vi "EstimateStates.vi"(8 "error in (no error)":errorcluster, 10 "Vessel in":refnum<class "Vessel.lvclass">, 11 "Kalman Filter in":refnum<class "Kalman Filter.lvclass">) -> (0 "error out":errorcluster, 2 "Vessel out":refnum<class "Vessel.lvclass">, 3 "Kalman Filter out":refnum<class "Kalman Filter.lvclass">)   [LabVIEW 2014, in "Observer Library.lvlib" / "Kalman Filter.lvclass"]
uses:
  Kalman Filter.lvclass
  ROV/Vessel.lvclass
  <vilib>/Analysis/Matrix/Numeric/Conversions/Matrix To Array - RM.vi
  <vilib>/imath/engines/lvmath2/RunTimeEngine/IndexRead/NIMS V(S).vi
  <instcachedir>/0/NIMS V(S)_0488751826AF41519A22953C041130DC.lvgen/NIMS V(S)_0488751826AF41519A22953C041130DC_000.vi
  <vilib>/imathl/engines/lvmath/Functions/Error Handling/Create Error.vi
  <vilib>/imath/engines/lvmath2/RunTimeEngine/IndexReplace/NIMS V(S)=S.vi
  <instcachedir>/0/NIMS V(S)=S_2D52C4EC15D8415E870AEE69FB516CCA.lvgen/NIMS V(S)=S_2D52C4EC15D8415E870AEE69FB516CCA_000.vi
  <vilib>/imath/engines/lvmath2/RunTimeEngine/BuiltInFunctions/mod/NIMS_mod_no_size_check.vi
  <instcachedir>/0/NIMS_mod_no_size_check_5393E3382FD241D281EEB71DA286C65B.lvgen/NIMS_mod_no_size_check_5393E3382FD241D281EEB71DA286C65B_001.vi
  <vilib>/imath/engines/lvmath2/RunTimeEngine/RangeToken/NIMS_Range.vi
  <instcachedir>/0/NIMS_Range_9BCE657718DF4976A877346C61F22738.lvgen/NIMS_Range_9BCE657718DF4976A877346C61F22738_000.vi
  <vilib>/imath/engines/lvmath2/RunTimeSupport/NIMS_Error if Not Equal.vi
  <instcachedir>/0/NIMS_Error if Not Equal_8A0E9F659B9142D69417CC259581C4FD.lvgen/NIMS_Error if Not Equal_8A0E9F659B9142D69417CC259581C4FD_001.vi
  <vilib>/imath/engines/lvmath2/RunTimeEngine/IndexRead/NIMS M(V,$).vi
  <instcachedir>/0/NIMS M(V,$)_21A5155762F74C04AE4EA67BEE0D3EF5.lvgen/NIMS M(V,$)_21A5155762F74C04AE4EA67BEE0D3EF5_004.vi
  <vilib>/imath/engines/lvmath2/RunTimeEngine/ErrorHandling/NIMS_Create Error From Enums.vi
  <vilib>/imath/engines/lvmath2/RunTimeEngine/ArithmeticOperatorToken/NIMS_ArithmeticOperator_multmx.vi
  <instcachedir>/0/NIMS_ArithmeticOperator_multmx_CE3986B82B8C4E94A31593A7EF82383B.lvgen/NIMS_ArithmeticOperator_multmx_CE3986B82B8C4E94A31593A7EF82383B_004.vi
  <vilib>/imath/engines/lvmath2/RunTimeEngine/ArithmeticOperatorToken/NIMS_ArithmeticOperator_plus.vi
  <instcachedir>/0/NIMS_ArithmeticOperator_plus_48D6EAACA5D645B09F7EC9C016C2DEA8.lvgen/NIMS_ArithmeticOperator_plus_48D6EAACA5D645B09F7EC9C016C2DEA8_003.vi
  <vilib>/imath/engines/lvmath2/RunTimeEngine/BuiltInFunctions/inv/NIMS_inv(GM).vi
  <instcachedir>/0/NIMS_inv(GM)_A6DF8FE880224208AACFE4CF9F659502.lvgen/NIMS_inv(GM)_A6DF8FE880224208AACFE4CF9F659502_000.vi
  <vilib>/imath/engines/lvmath2/RunTimeEngine/ArithmeticOperatorToken/NIMS_ArithmeticOperator_minus.vi
  <instcachedir>/0/NIMS_ArithmeticOperator_minus_39C0593E74DA4138ACA2AB742906488D.lvgen/NIMS_ArithmeticOperator_minus_39C0593E74DA4138ACA2AB742906488D_009.vi
  <vilib>/imath/engines/lvmath2/RunTimeEngine/ArithmeticOperatorToken/NIMS_ArithmeticOperator_multmx(M,CV).vi
  <instcachedir>/0/NIMS_ArithmeticOperator_multmx(M,CV)_787B4652E60B4C52835A7FB23671E425.lvgen/NIMS_ArithmeticOperator_multmx(M,CV)_787B4652E60B4C52835A7FB23671E425_000.vi
  <instcachedir>/0/NIMS_ArithmeticOperator_minus_39C0593E74DA4138ACA2AB742906488D.lvgen/NIMS_ArithmeticOperator_minus_39C0593E74DA4138ACA2AB742906488D_002.vi
  <vilib>/imath/engines/lvmath2/RunTimeEngine/IndexRead/NIMS M(S).vi
  <instcachedir>/0/NIMS M(S)_B826C018497E4940AE96BD27B540B6FB.lvgen/NIMS M(S)_B826C018497E4940AE96BD27B540B6FB_000.vi
  <vilib>/imath/engines/lvmath2/RunTimeEngine/IndexReplace/NIMS M(S)=S.vi
  <instcachedir>/0/NIMS M(S)=S_D871EE7B27E5455586ED06C330670F09.lvgen/NIMS M(S)=S_D871EE7B27E5455586ED06C330670F09_001.vi
  <vilib>/imath/engines/lvmath2/RunTimeEngine/IndexRead/NIMS M(R2).vi
  <instcachedir>/0/NIMS M(R2)_287818D58BD74005B29FE73CE7602B1A.lvgen/NIMS M(R2)_287818D58BD74005B29FE73CE7602B1A_000.vi
  <vilib>/imath/engines/lvmath2/RunTimeEngine/BuiltInFunctions/atan2/NIMS_atan2.vi
  <instcachedir>/0/NIMS_atan2_A91AA4A7D42247EDBE8F76DB99AF04A4.lvgen/NIMS_atan2_A91AA4A7D42247EDBE8F76DB99AF04A4_000.vi
  <vilib>/imath/engines/lvmath2/RunTimeEngine/NodeEndStatement/NIMS_NodeEndStatement_Get Vector.vi
  <instcachedir>/0/NIMS_NodeEndStatement_Get Vector_00D1625602D843AD9D7EC134A9EC13A2.lvgen/NIMS_NodeEndStatement_Get Vector_00D1625602D843AD9D7EC134A9EC13A2_001.vi
  <vilib>/imath/engines/lvmath/Functions/Error Handling/MergeErrorsWrapper.vi
  <vilib>/imath/engines/lvmath2/RunTimeEngine/NodeEndStatement/NIMS_NodeEndStatement_Output.vi
  <instcachedir>/0/NIMS_NodeEndStatement_Output_53EC0D466D134D7ABD903AC30B43404B.lvgen/NIMS_NodeEndStatement_Output_53EC0D466D134D7ABD903AC30B43404B_002.vi
  <instcachedir>/0/NIMS_NodeEndStatement_Output_53EC0D466D134D7ABD903AC30B43404B.lvgen/NIMS_NodeEndStatement_Output_53EC0D466D134D7ABD903AC30B43404B_005.vi
  <instcachedir>/0/NIMS_NodeEndStatement_Output_53EC0D466D134D7ABD903AC30B43404B.lvgen/NIMS_NodeEndStatement_Output_53EC0D466D134D7ABD903AC30B43404B_001.vi
  <vilib>/imath/engines/lvmath2/RunTimeEngine/ErrorHandling/NIMS_Finalize Error.vi
  Supervisor/Supervisor.lvclass
  <vilib>/Analysis/Matrix/NI_Matrix.lvlib
panel:
  out "H out":i32[][](array[numeric])
  in  "P_bar":dbl[][](array[numeric])=[[1.0, 0.0, 0.0, 0.0, 0.0, 0.0, 0.0, 0.0, 0.0, 0.0, 0.0, 0.0, 0.0, 0.0, 0.0, 0.0, 0.0, 0.0], [0.0, 0.0, 0.0, 0.0, 0.0, 0.0, 0.0, 0.0, 0.0, 0.0, 0.0, 0.0, 0.0, 0.0, 0.0, 0.0, 0.0, 0.0], [0.0, 0.0, 0.0, 0.0, 0.0, 0.0, 0.0, 0.0, 0.0, 0.0, 0.0, 0.0, 0.0, 0.0, 0.0, 0.0, 0.0, 0.0], [0.0, 0.0, 0.0, 0.0, 0.0, 0.0, 0.0, 0.0, 0.0, 0.0, 0.0, 0.0, 0.0, 0.0, 0.0, 0.0, 0.0, 0.0], [0.0, 0.0, 0.0, 0.0, 0.0, 0.0, 0.0, 0.0, 0.0, 0.0, 0.0, 0.0, 0.0, 0.0, 0.0, 0.0, 0.0, 0.0], [0.0, 0.0, 0.0, 0.0, 0.0, 0.0, 0.0, 0.0, 0.0, 0.0, 0.0, 0.0, 0.0, 0.0, 0.0, 0.0, 0.0, 0.0], [0.0, 0.0, 0.0, 0.0, 0.0, 0.0, 0.0, 0.0, 0.0, 0.0, 0.0, 0.0, 0.0, 0.0, 0.0, 0.0, 0.0, 0.0], [0.0, 0.0, 0.0, 0.0, 0.0, 0.0, 0.0, 0.0, 0.0, 0.0, 0.0, 0.0, 0.0, 0.0, 0.0, 0.0, 0.0, 0.0], [0.0, 0.0, 0.0, 0.0, 0.0, 0.0, 0.0, 0.0, 0.0, 0.0, 0.0, 0.0, 0.0, 0.0, 0.0, 0.0, 0.0, 0.0], [0.0, 0.0, 0.0, 0.0, 0.0, 0.0, 0.0, 0.0, 0.0, 0.0, 0.0, 0.0, 0.0, 0.0, 0.0, 0.0, 0.0, 0.0], [0.0, 0.0, 0.0, 0.0, 0.0, 0.0, 0.0, 0.0, 0.0, 0.0, 0.0, 0.0, 0.0, 0.0, 0.0, 0.0, 0.0, 0.0], [0.0, 0.0, 0.0, 0.0, 0.0, 0.0, 0.0, 0.0, 0.0, 0.0, 0.0, 0.0, 0.0, 0.0, 0.0, 0.0, 0.0, 0.0], [0.0, 0.0, 0.0, 0.0, 0.0, 0.0, 0.0, 0.0, 0.0, 0.0, 0.0, 0.0, 0.0, 0.0, 0.0, 0.0, 0.0, 0.0], [0.0, 0.0, 0.0, 0.0, 0.0, 0.0, 0.0, 0.0, 0.0, 0.0, 0.0, 0.0, 0.0, 0.0, 0.0, 0.0, 0.0, 0.0], [0.0, 0.0, 0.0, 0.0, 0.0, 0.0, 0.0, 0.0, 0.0, 0.0, 0.0, 0.0, 0.0, 0.0, 0.0, 0.0, 0.0, 0.0], [0.0, 0.0, 0.0, 0.0, 0.0, 0.0, 0.0, 0.0, 0.0, 0.0, 0.0, 0.0, 0.0, 0.0, 0.0, 0.0, 0.0, 0.0], [0.0, 0.0, 0.0, 0.0, 0.0, 0.0, 0.0, 0.0, 0.0, 0.0, 0.0, 0.0, 0.0, 0.0, 0.0, 0.0, 0.0, 0.0], [0.0, 0.0, 0.0, 0.0, 0.0, 0.0, 0.0, 0.0, 0.0, 0.0, 0.0, 0.0, 0.0, 0.0, 0.0, 0.0, 0.0, 0.0]]
  out "K":dbl[][](array[numeric])
  out "i":dbl
  out "b_dir":dbl
  out "Bias [N]":T1(graph)
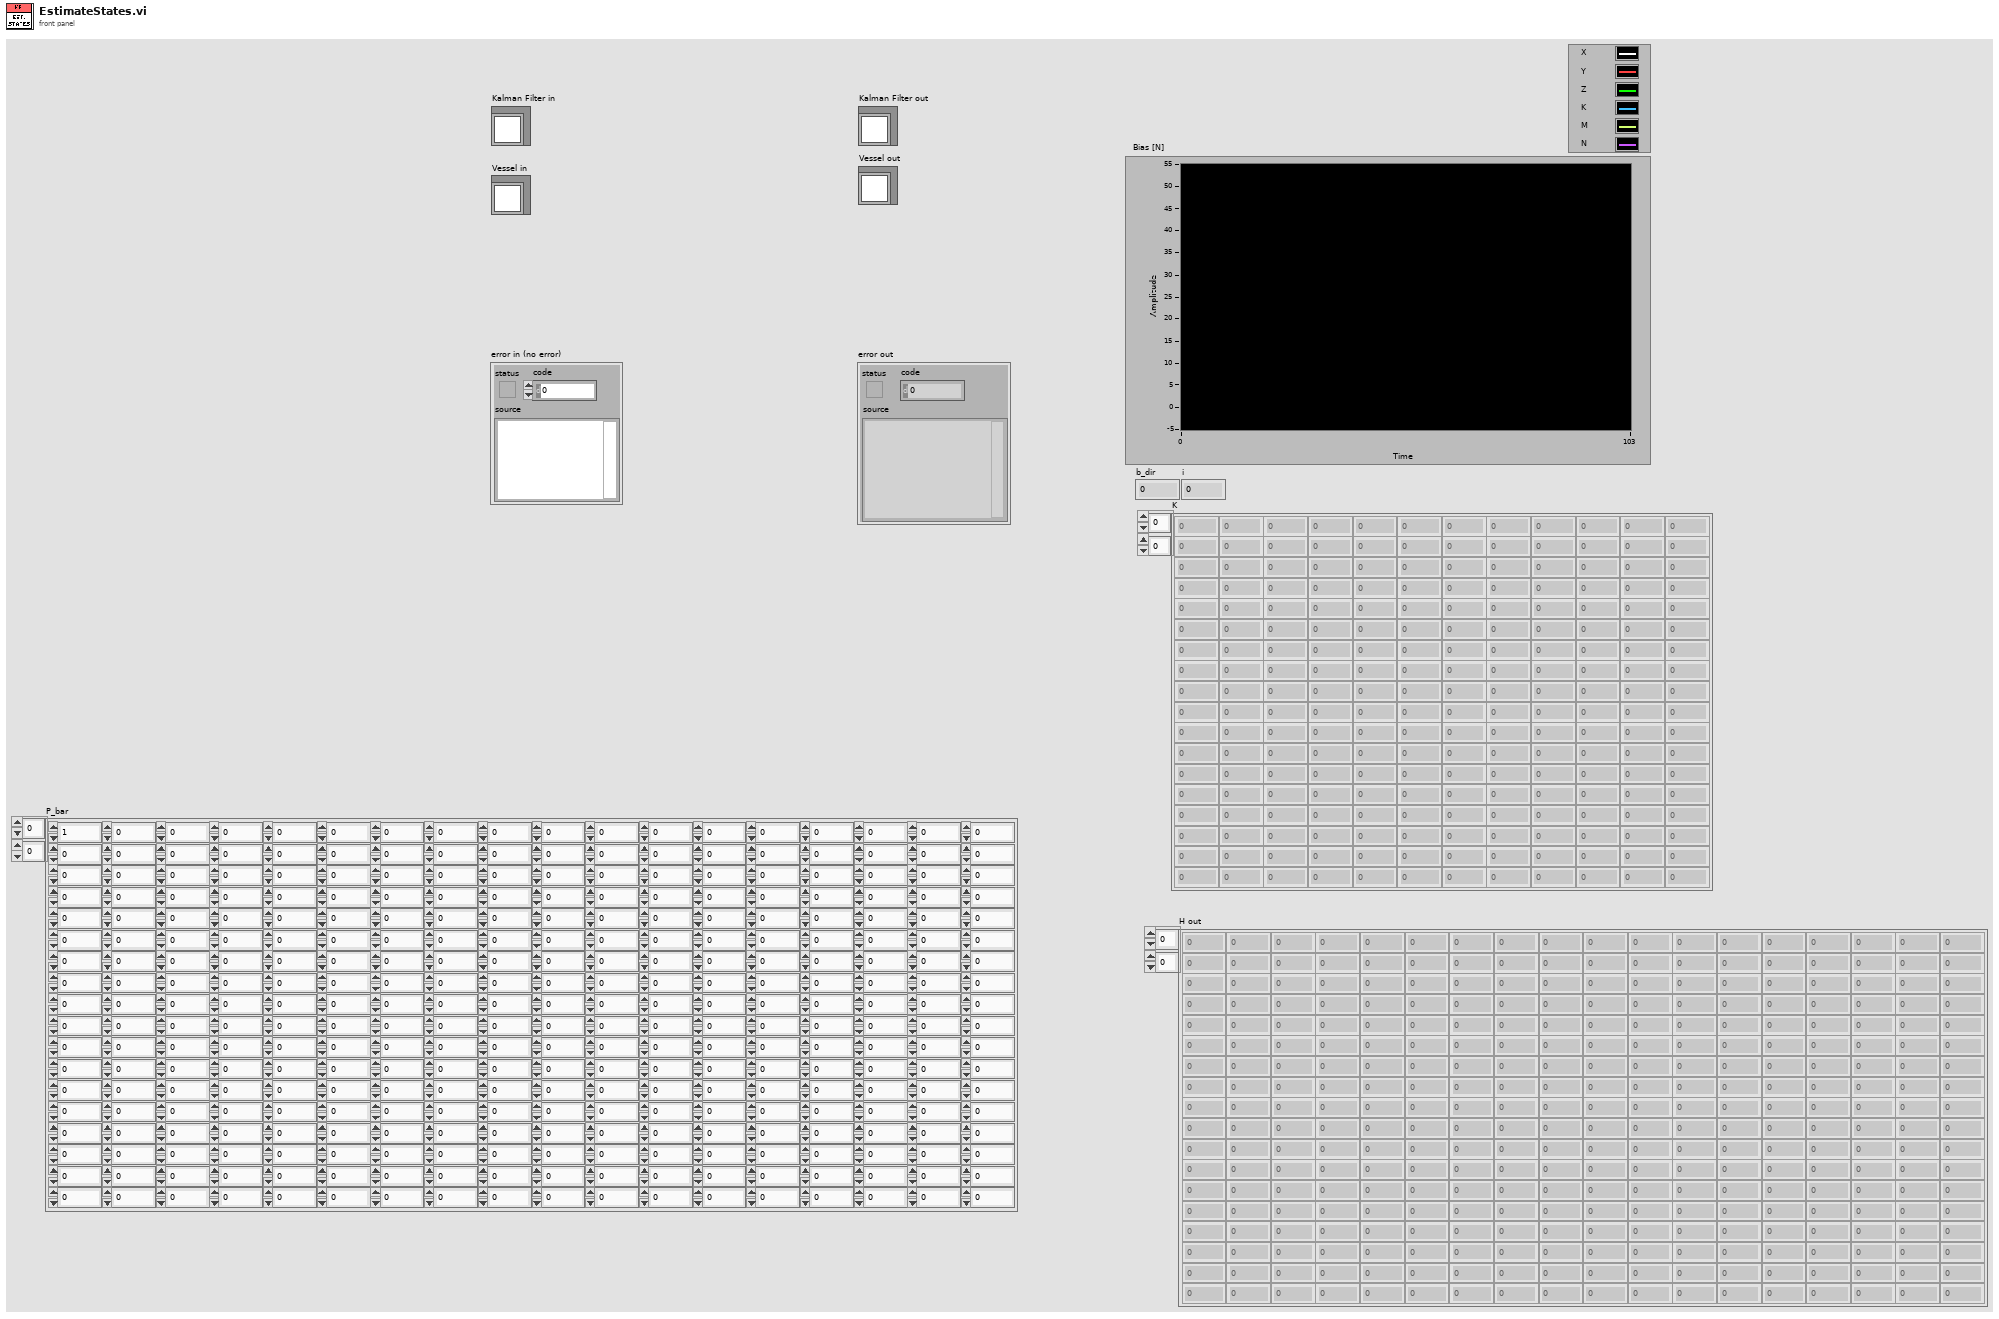
[diagram p1: front panel]
types:
  T1 = cluster{"b_hat[0]":dbl, "b_hat[1]":dbl, "b_hat[2]":dbl, "b_hat[3]":dbl, "b_hat[4]":dbl, "b_hat[5]":dbl, "b_hat[6]":dbl, "b_hat[7]":dbl, "b_hat[8]":dbl}
  T2 = typedef "NI_Matrix.lvlib/RealMatrix.ctl" = dbl[][]
  T3 = cluster{"Measured":cluster{"Eta":dbl[], "Nu":dbl[], "Eta Dot":dbl[], "Nu Dot":dbl[]}, "Estimated":cluster{"Eta":dbl[], "Nu":dbl[], "Eta Dot":dbl[], "Nu Dot":dbl[]}, "Desired":cluster{"Eta":dbl[], "Nu":dbl[], "Eta Dot":dbl[], "Nu Dot":dbl[]}, "Previous Desired":cluster{"Eta":dbl[], "Nu":dbl[], "Eta Dot":dbl[], "Nu Dot":dbl[]}, "tau":dbl[], "Altitude":cluster{"Measured":dbl, "Estimated":dbl, "Desired":dbl, "Previous Desired":dbl, "Approximated":dbl, "grad F":dbl[]}, "rpm":dbl[], "Attitude":cluster{"Theta Measured":dbl[], "Theta Estimated":dbl[], "Omega Measured":dbl[], "Omega Estimated":dbl[], "Gyro Bias":dbl[]}}
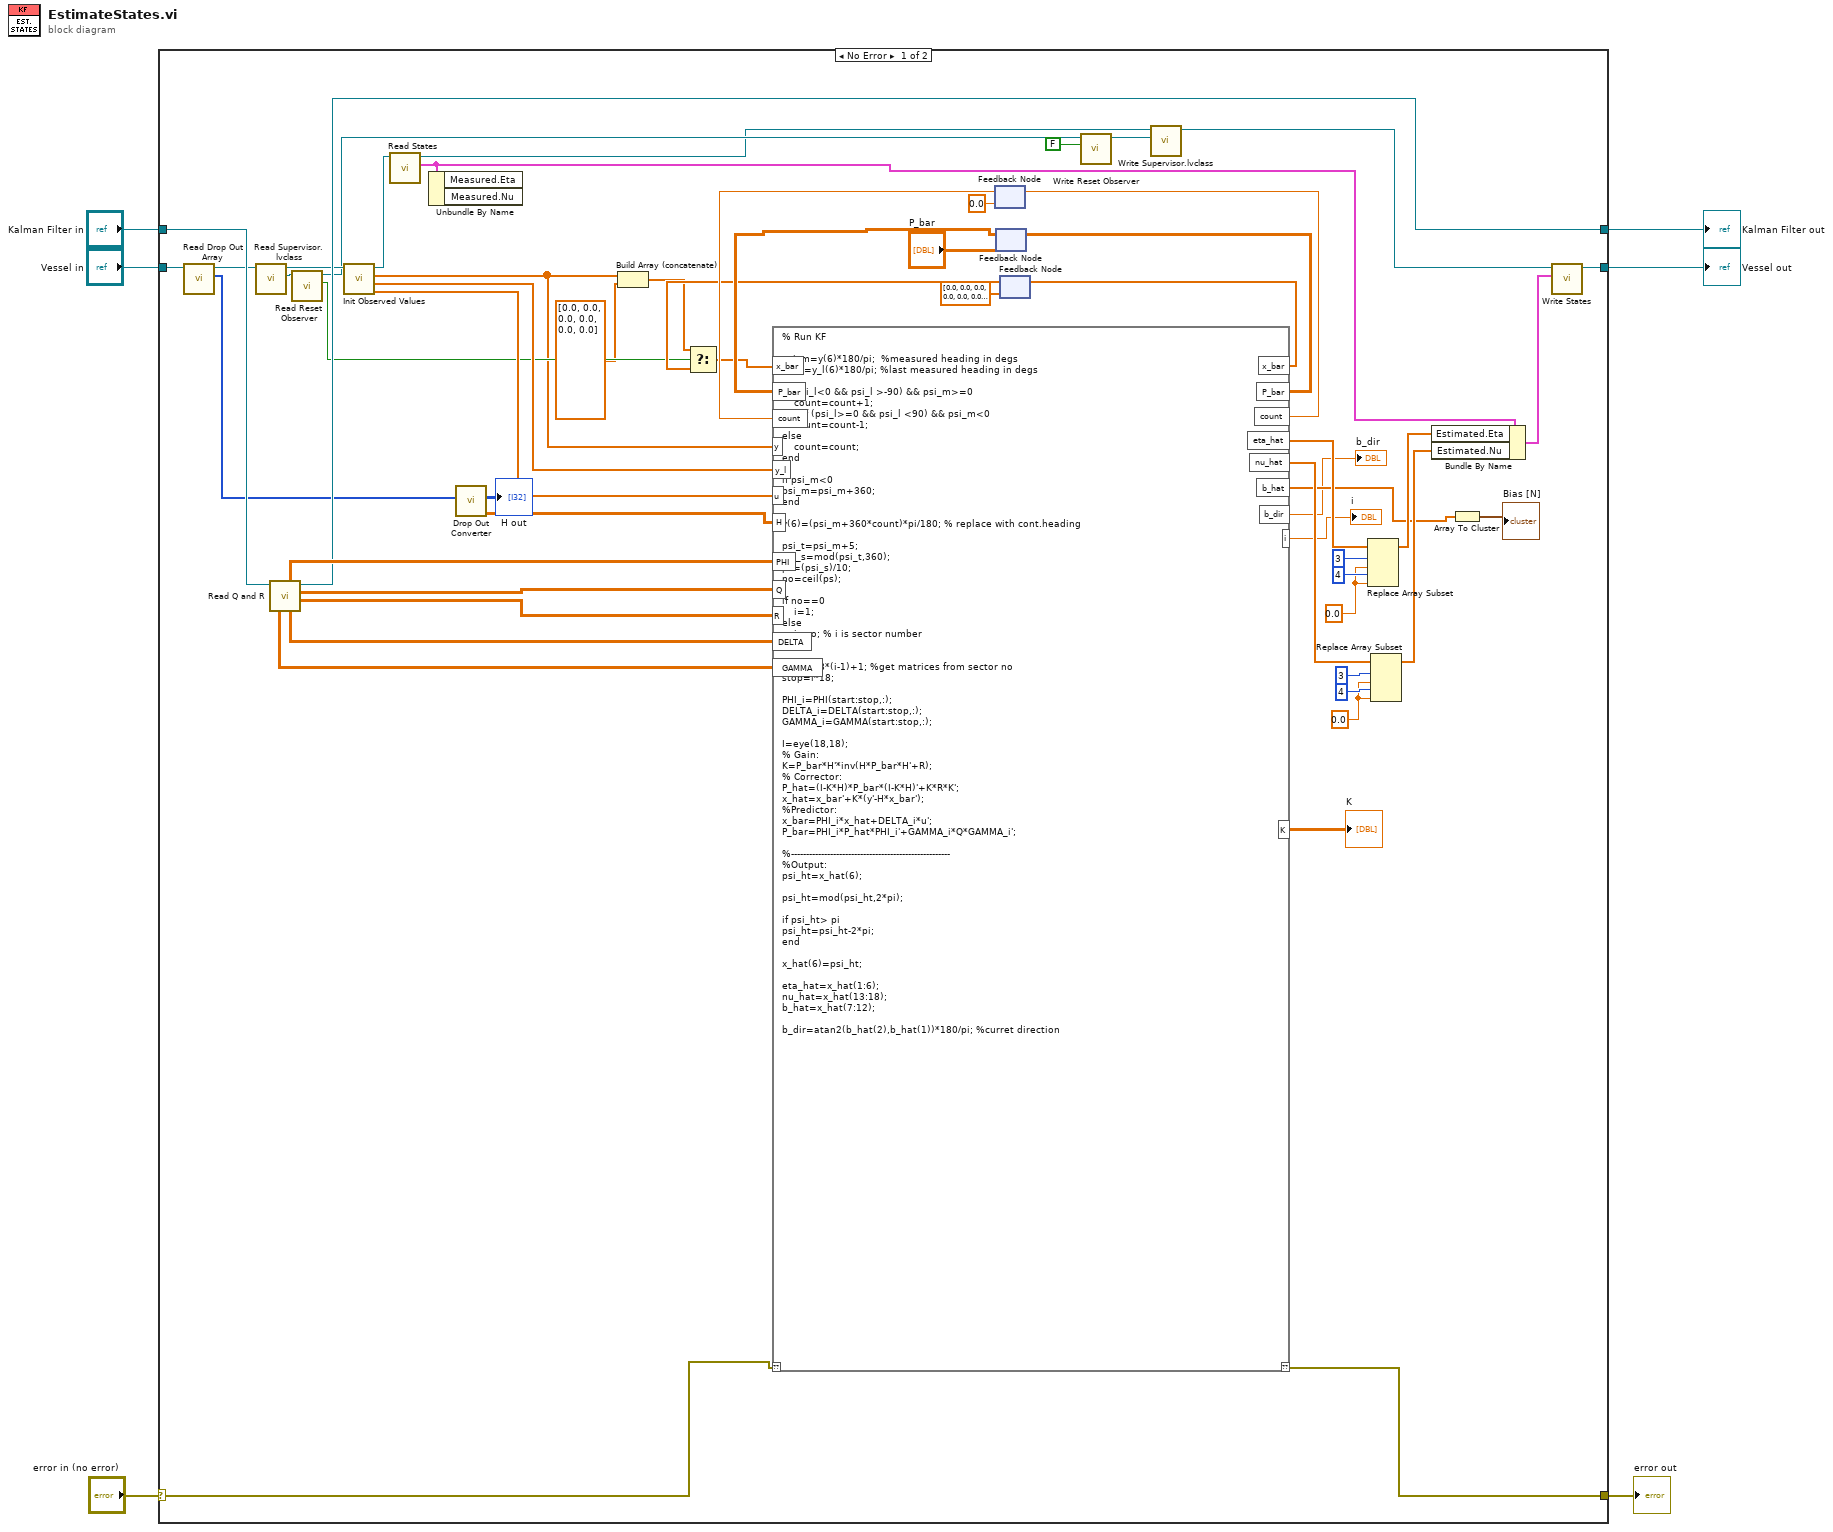
[diagram p0: block diagram]
diagram:
  n1 = case shown="No Error" "error in (no error)" {
    selector: "error in (no error)" -> [w14 w861]
    tunnel: [w13 w861] -> w5
    tunnel: "Vessel in" -> [w22 w862]
    tunnel: "Kalman Filter in" -> [w62 w863]
    tunnel: [w48 w863] -> w3
    tunnel: [w50 w862] -> w1
    frame No Error {
      w39 = 0.0 ("new element/subarray")
      w42 = 0.0 ("new element/subarray")
      n2 = call-dynamic "Read Drop Out Array.vi"("Vessel in"=w22) -> ("Drop Out Array"=w20:i32[], "Vessel out"=w21:refnum<class "Vessel.lvclass">)  [unwired: 8 in, 1 out]
      n3 = call "Read Supervisor.lvclass.vi"("Vessel in"=w21) -> ("Supervisor.lvclass"=w34:refnum<class "Supervisor.lvclass">, "Vessel out"=w35:refnum<class "Vessel.lvclass">)  [unwired: 8 in, 1 out]
      n4 = call-dynamic "Read Q and R.vi"("Kalman Filter in"=w62) -> ("R Out"=w54:T2, "Q Out"=w55:T2, "Kalman Filter out"=w48:refnum<class "Kalman Filter.lvclass">, "DELTA out"=w53:T2, "PHI out"=w51:T2, "GAMMA out"=w52:T2)  [unwired: 4 in, 1 out]
      n5 = call-dynamic "Read Reset Observer.vi"("Supervisor in"=w34) -> ("Reset Observer"=w23:bool, "Supervisor out"=w31:refnum<class "Supervisor.lvclass">)  [unwired: 8 in, 1 out]
      n6 = call "Init Observed Values.vi"("Vessel in"=w35) -> ("tau"=w56:dbl[], "y_l"=w57:dbl[], "y"=w19:dbl[], "Vessel out"=w30:refnum<class "Vessel.lvclass">)  [unwired: 7 in]
      n7 = call-dynamic "Read States.vi"("Vessel in"=w30) -> ("States"=w27:T3, "Vessel out"=w29:refnum<class "Vessel.lvclass">)  [unwired: 8 in, 1 out]
      n8 = Unbundle By Name(w27) -> ()  [unwired: 2 out]
      n9 = call "Drop Out Converter.vi"("Drop out in"=w20) -> ("H"=w16:T2, "H out"=→"H out":i32[][])  [unwired: 9 in]
      n10 = Build Array (concatenate)(w19, dbl[] [0.0, 0.0, 0.0, 0.0, 0.0, 0.0]) -> (w17:dbl[])
      n11 = feedback #1(0.0 ("count")) -> (w58:dbl)
      n12 = feedback #2("P_bar") -> (w26:dbl[][])
      n13 = feedback #3(dbl[] [0.0, 0.0, 0.0, 0.0, 0.0, 0.0, 0.0, 0.0, 0.0, 0.0, 0.0, 0.0, 0.0, 0.0, 0.0, 0.0, 0.0, 0.0] ("x_bar")) -> (w25:dbl[])
      n14 = Select(t=w17, s=w23, f=w25) -> (s? t:f=w24:dbl[])
      n15 = mathscript code="% Run KF\n\npsi_m=y(6)*180/pi;  %measured heading in degs\npsi_l=y_l(6)*180/pi; %last measured heading in degs\n\nif (psi_l<0 && psi_l >-90) && psi_m>=0\n    count=count+1;    \nelseif (psi_l>=0 && psi_l <90) && psi_m<0\n    count=count-1;\nelse    \n    count=count;\nend\n\nif psi_m<0\npsi_m=psi_m+360;\nend\n\ny(6)=(psi_m+360*count)*pi/180; % replace with cont.heading \n\npsi_t=psi_m+5;\npsi_s=mod(psi_t,360);\nps=(psi_s)/10;\nno=ceil(ps);\n\nif no==0\n    i=1;\nelse\n    i=no; % i is sector number\nend\n\nstart=18*(i-1)+1; %get matrices from sector no\nstop=i*18;\n\nPHI_i=PHI(start:stop,:);\nDELTA_i=DELTA(start:stop,:);\nGAMMA_i=GAMMA(start:stop,:);\n\nI=eye(18,18);\n% Gain:\nK=P_bar*H'*inv(H*P_bar*H'+R);\n% Corrector:\nP_hat=(I-K*H)*P_bar*(I-K*H)'+K*R*K';\nx_hat=x_bar'+K*(y'-H*x_bar');\n%Predictor:\nx_bar=PHI_i*x_hat+DELTA_i*u'; \nP_bar=PHI_i*P_hat*PHI_i'+GAMMA_i*Q*GAMMA_i';\n\n%-----------------------------------------------------\n%Output:\npsi_ht=x_hat(6);\n\npsi_ht=mod(psi_ht,2*pi);\n\nif psi_ht> pi\npsi_ht=psi_ht-2*pi;\nend\n\nx_hat(6)=psi_ht;\n\neta_hat=x_hat(1:6);\nnu_hat=x_hat(13:18);\nb_hat=x_hat(7:12);\n\nb_dir=atan2(b_hat(2),b_hat(1))*180/pi; %curret direction"("??"=w14, "P_bar"=w26, "x_bar"=w24, "PHI"=w51, "DELTA"=w53, "GAMMA"=w52, "Q"=w55, "R"=w54, "H"=w16, "y"=w19, "u"=w56, "y_l"=w57, "count"=w58) -> ("??"=w13:errorcluster, "P_bar"=w60:dbl[][], "x_bar"=w61:dbl[], "nu_hat"=w38:dbl[], "b_hat"=w12:dbl[], "b_dir"=→"b_dir":dbl, "i"=→"i":dbl, "count"=w59:dbl, "eta_hat"=w15:dbl[], "K"=→"K":dbl[][])
      n16 = feedback-in #1(w59) -> ()
      n17 = feedback-in #2(w60) -> ()
      n18 = feedback-in #3(w61) -> ()
      n19 = call-dynamic "Write Reset Observer.vi"("Reset Observer"=FALSE, "Supervisor in"=w31) -> ("Supervisor out"=w33:refnum<class "Supervisor.lvclass">)  [unwired: 8 in, 1 out]
      n20 = call "Write Supervisor.lvclass.vi"("Supervisor.lvclass"=w33, "Vessel in"=w29) -> ("Vessel out"=w28:refnum<class "Vessel.lvclass">)  [unwired: 8 in, 1 out]
      n21 = Replace Array Subset(array=w15, new element #1=w42, index #1=3 ("index"), new element #2=w42, index #2=4 ("index")) -> (w37:dbl[])
      n22 = Replace Array Subset(array=w38, new element #1=w39, index #1=3 ("index"), new element #2=w39, index #2=4 ("index")) -> (w36:dbl[])
      n23 = Bundle By Name(cluster=w27, "Estimated.Eta"=w37, "Estimated.Nu"=w36) -> (w49:T3)
      n24 = Array To Cluster(array=w12) -> (cluster=→"Bias [N]":T1)
      n25 = call-dynamic "Write States.vi"("States"=w49, "Vessel in"=w28) -> ("Vessel out"=w50:refnum<class "Vessel.lvclass">)  [unwired: 8 in, 1 out]
    }
    frame Error {
    }
  }
  "error out" <- w5
  "Kalman Filter out" <- w3
  "Vessel out" <- w1
